vi "Location Routine.vi"(8 "error in":errorcluster, 11 "Refnum in":refnum<k20>) -> (0 "error out":errorcluster, 3 "Refnum out":refnum<k20>)   [LabVIEW 2012]
uses:
  <vilib>/Platform/TimedLoop/XDataNode/timing_clust.ctl
  <vilib>/Platform/TimedLoop/XDataNode/nitl_modes.ctl
  <vilib>/Platform/TimedLoop/XDataNode/wakeup.ctl
  Globals.vi
  <vilib>/platform/TimedLoop/XDataNode/XDataNode.xnode
  <vilib>/Platform/TimedLoop/XDataNode/XDNodeRunTimeDep.lvlib
panel:
  in  "stop":bool
  out "Waveform Chart":cluster{dbl, dbl}(graph)
  out "read buffer":string
  out "Full packet?":bool
  out "Heading (deg)":dbl
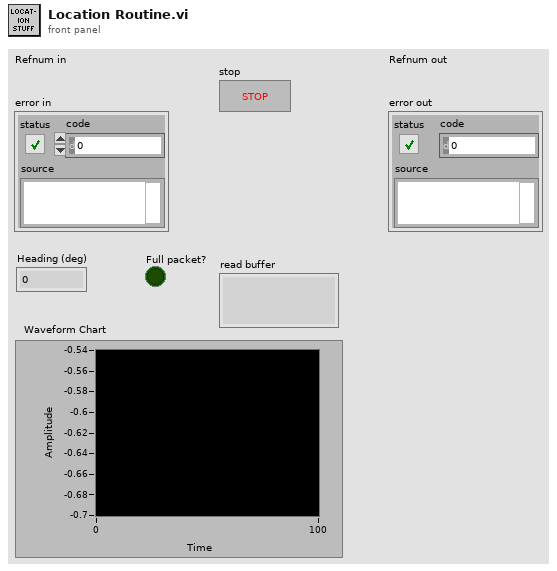
[diagram p1: front panel]
types:
  T1 = typedef "XDNodeRunTimeDep.lvlib/timing_clust.ctl" = cluster{"Expected End [f-1]":u64, "Actual End [f-1]":u64, "Finished Late? [f-1]":bool, "Expected End [i-1]":u64, "Actual End [i-1]":u64, "Finished Late? [i-1]":bool, "Expected Start [i]":u64, "Actual Start [i]":u64, "Expected Start [f]":u64, "Actual Start [f]":u64, "Source Name":string, "Structure Name":string, "Period":i64, "Deadline":i64, "Offset":i64, "Start":i64, "Priority":i32, "Timeout":i32, "Mode":T2, "Wakeup Reason":T3, "Error":errorcluster, "Source Type":string, "Secondary Source Type":string, "Global End Time":u64, "Global Start Time":u64, "Frame Duration":u64, "Iteration Duration":u64, "Assigned CPU":i32, "I/O Scan Engine Mode":u32}
  T2 = typedef "XDNodeRunTimeDep.lvlib/nitl_modes.ctl" = enum32{"No Change", "Process missed periods, maintain original phase", "Discard missed periods, maintain original phase", "Process missed periods, ignore original phase", "Discard missed periods, ignore original phase"}
  T3 = typedef "XDNodeRunTimeDep.lvlib/wakeup.ctl" = enum32{"Normal", "Aborted", "Asynchronous wakeup", "Timing source error", "Timed loop error", "Timeout"}
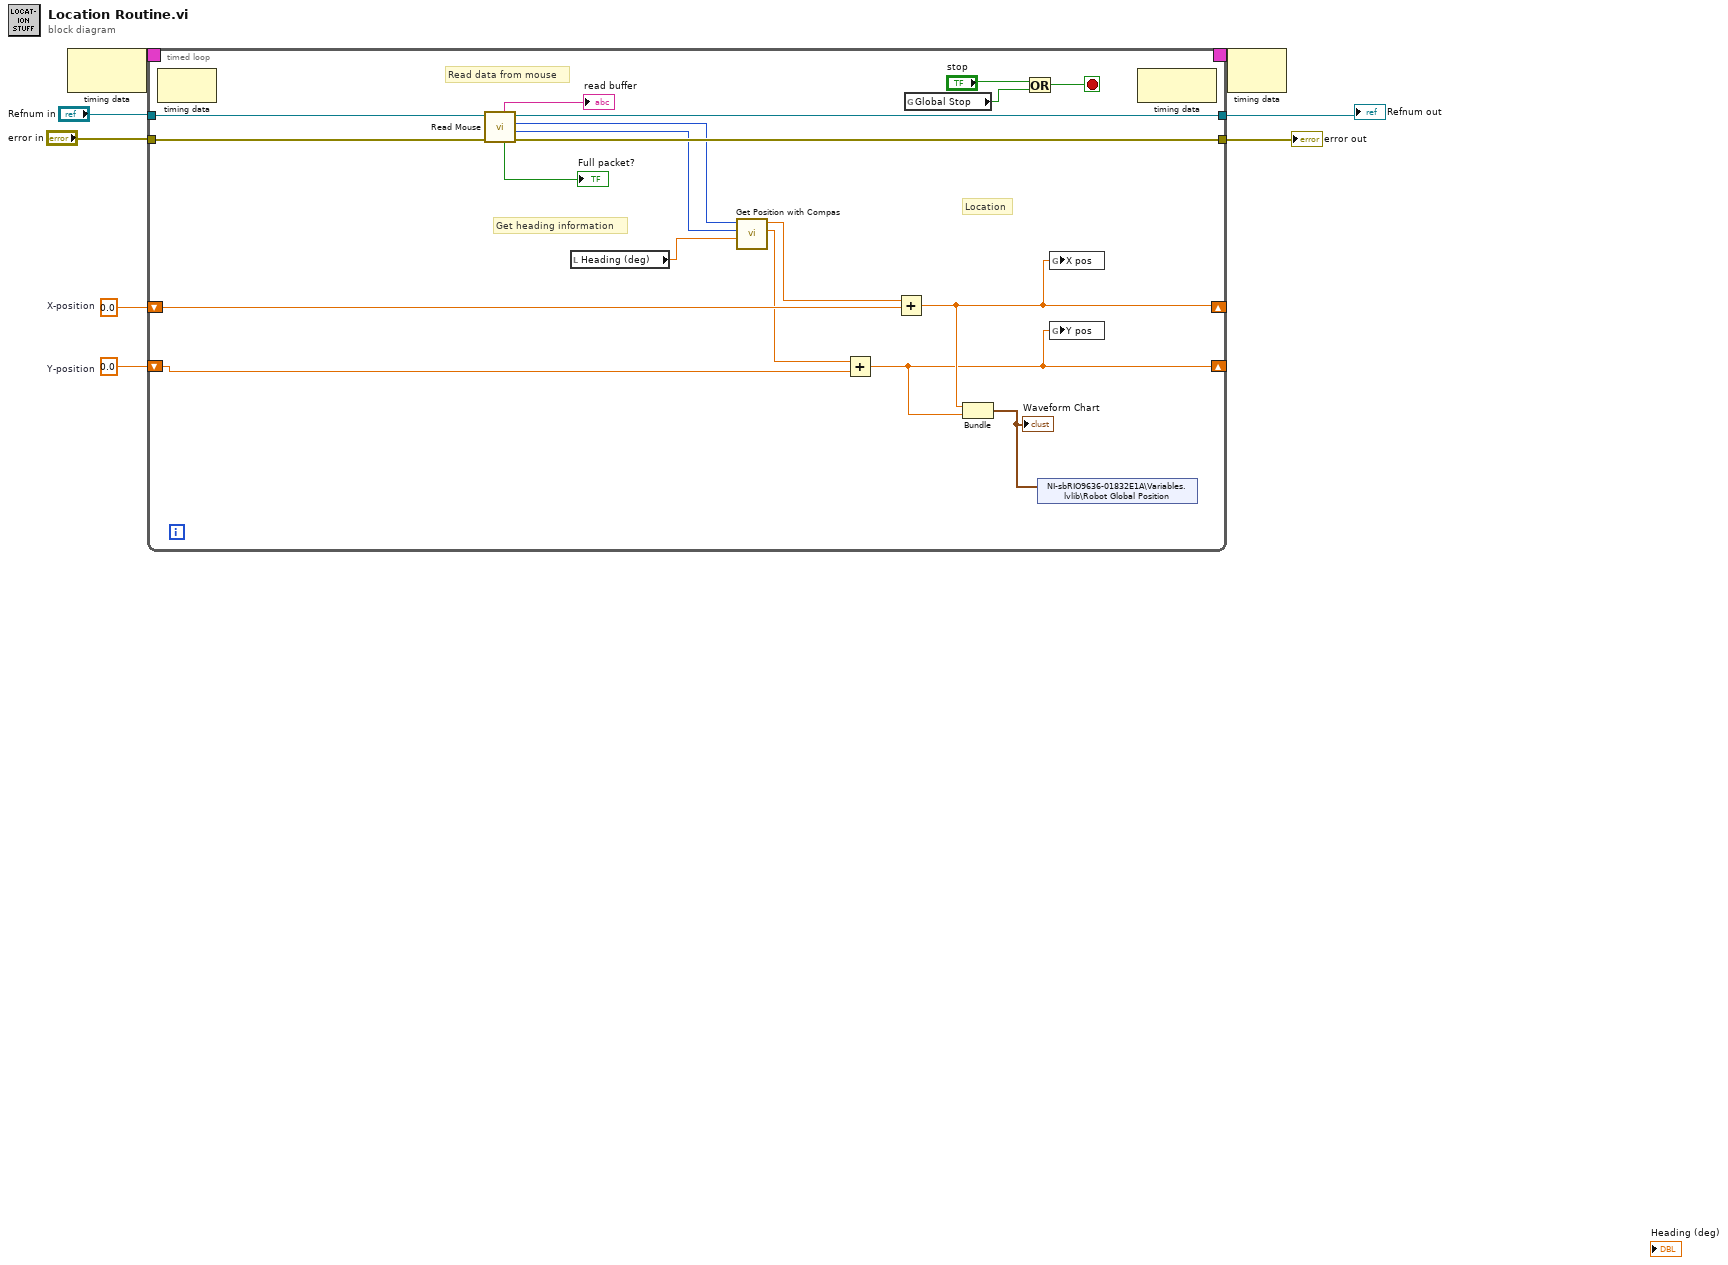
[diagram p0: block diagram]
diagram:
  w5 = 0.0  # Y-position
  w6 = 0.0  # X-position
  n1 = node-c288() -> (w4:T1)  [unwired: 1 in]
  n2 = timed-loop {
    tunnel: [w26] -> w1
    tunnel: "error in" -> [w24]
    tunnel: "Refnum in" -> [w18]
    tunnel: [w23] -> w2
    shift-right: [w10] -> _
    shift-left: w6 -> [w16]
    shift-right: [w9] -> _
    shift-left: w5 -> [w15]
    timing: w4 -> [_]
    timing-out: [_] -> w3
    stop <- w27 stop-if-true
    # "Read data from mouse"
    # "Get heading information"
    # "Location"
    n3 = node-c288() -> ()  [unwired: 1 in, 1 out]
    n4 = call "Read Mouse.vi"("error in (no error)"=w24, "Refnum in"=w18) -> ("error out"=w26:errorcluster, "Delta y"=w19:i16, "Delta x"=w21:i16, "Refnum out"=w23:refnum<k20>, "Full packet?"=→"Full packet?":bool, "read buffer"=→"read buffer":string)  [unwired: 4 in]
    n5 = local read "Heading (deg)"() -> (w17:dbl)
    n6 = call "Get Position with Compas.vi"("Heading (deg)"=w17, "Delta y"=w19, "Delta x"=w21) -> ("y out"=w13:dbl, "x out"=w14:dbl)  [unwired: 7 in]
    n7 = Add(x=w13, y=w15) -> (x+y=w9:dbl)
    n8 = Add(x=w14, y=w16) -> (x+y=w10:dbl)
    n9 = global read "Globals.vi" "Global Stop"() -> (w11:bool)
    n10 = Bundle(w10, w9) -> (w12:cluster{dbl, dbl})  [unwired: 1 in]
    "Waveform Chart" <- w12
    n11 = Or(x="stop", y=w11) -> (x .or. y?=w27:bool)
    n12 = shared-variable "NI-sbRIO9636-01832E1A\\Variables.lvlib\\Robot Global Position"(w12) -> ()  [unwired: 1 in, 1 out]
    n13 = global write "Globals.vi" "X pos"(w10) -> ()
    n14 = global write "Globals.vi" "Y pos"(w9) -> ()
    n15 = node-c288() -> ()  [unwired: 1 in, 1 out]
  }
  "Refnum out" <- w2
  "error out" <- w1
  n16 = node-c288(w3) -> ()  [unwired: 1 out]
